vi "GetValuesFromRefs_USB7855R.vi"(6 "Array":cluster{"LSB Weight":u32, "Offset":i32}[](array[cluster]), 11 "ChangeonFly":T2) -> (3 "output cluster":T1)   [LabVIEW 2023]
uses:
  TypeDefs/ChangeOnFly.ctl
  User_Vi/Settings.vi
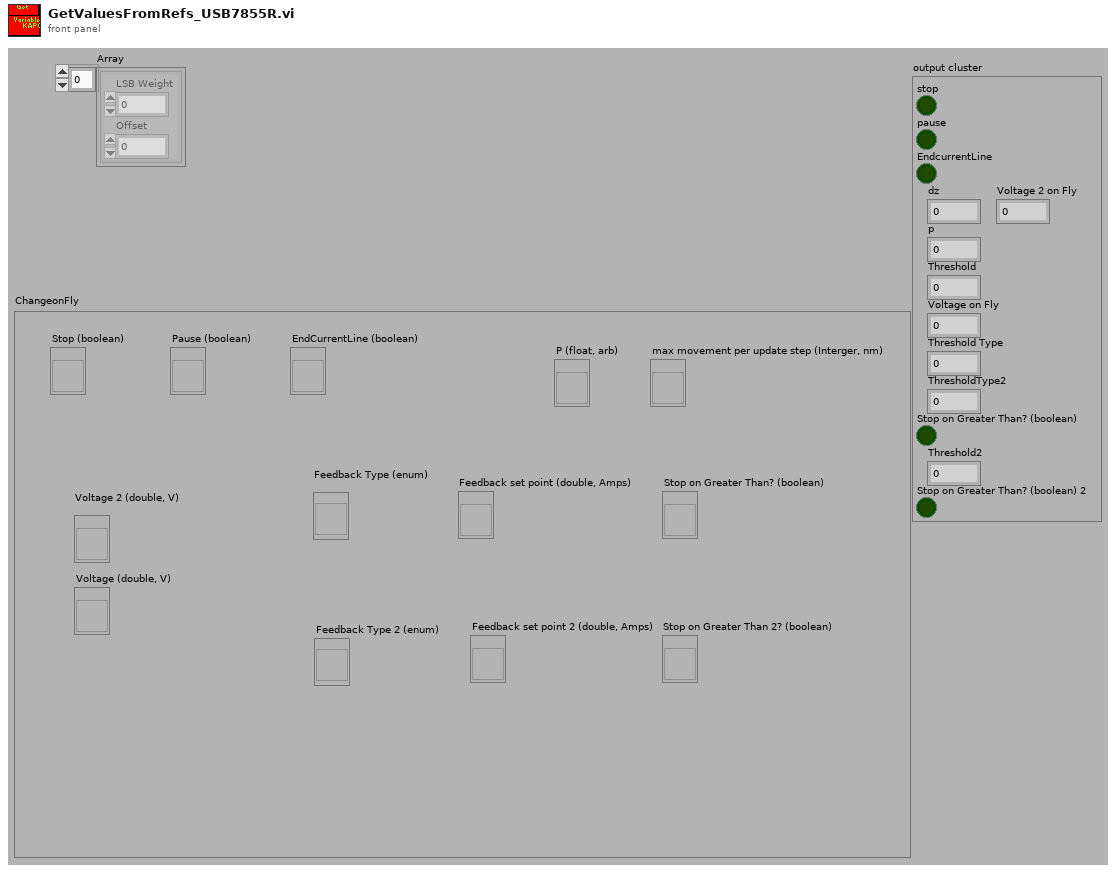
[diagram p1: front panel]
types:
  T1 = cluster{"stop":bool, "pause":bool, "EndcurrentLine":bool, "dz":i32, "p":fxp<+/-,32,1>, "Threshold":i32, "Voltage on Fly":i16, "Threshold Type":u8, "ThresholdType2":u8, "Stop on Greater Than? (boolean)":bool, "Threshold2":i32, "Stop on Greater Than? (boolean) 2":bool, "Voltage 2 on Fly":i16}
  T2 = typedef "ChangeOnFly.ctl" = cluster{"Stop (boolean)":refnum<vi>, "Pause (boolean)":refnum<vi>, "EndCurrentLine (boolean)":refnum<vi>, "max movement per update step (Interger, nm)":refnum<vi>, "P (float, arb)":refnum<vi>, "Feedback set point (double, Amps)":refnum<vi>, "Voltage (double, V)":refnum<vi>, "Feedback set point 2 (double, Amps)":refnum<vi>, "Stop on Greater Than 2? (boolean)":refnum<vi>, "Stop on Greater Than? (boolean)":refnum<vi>, "Voltage 2 (double, V)":refnum<vi>, "Feedback Type (enum)":refnum<vi>, "Feedback Type 2 (enum)":refnum<vi>}
  T3 = enum16{"AC Magnitude", "Current 1", "Current 2", "Phase"}
  T4 = enum16{"USB 7855 (AI)", "USB 7855 (AO)", "USB 7855 OEM (AI)", "USB 7855 OEM (AO)", "USB 7856  (AI)", "USB 7856 (AO)", "USB 7856 OEM (AI)", "USB 7856 OEM (AO)"}
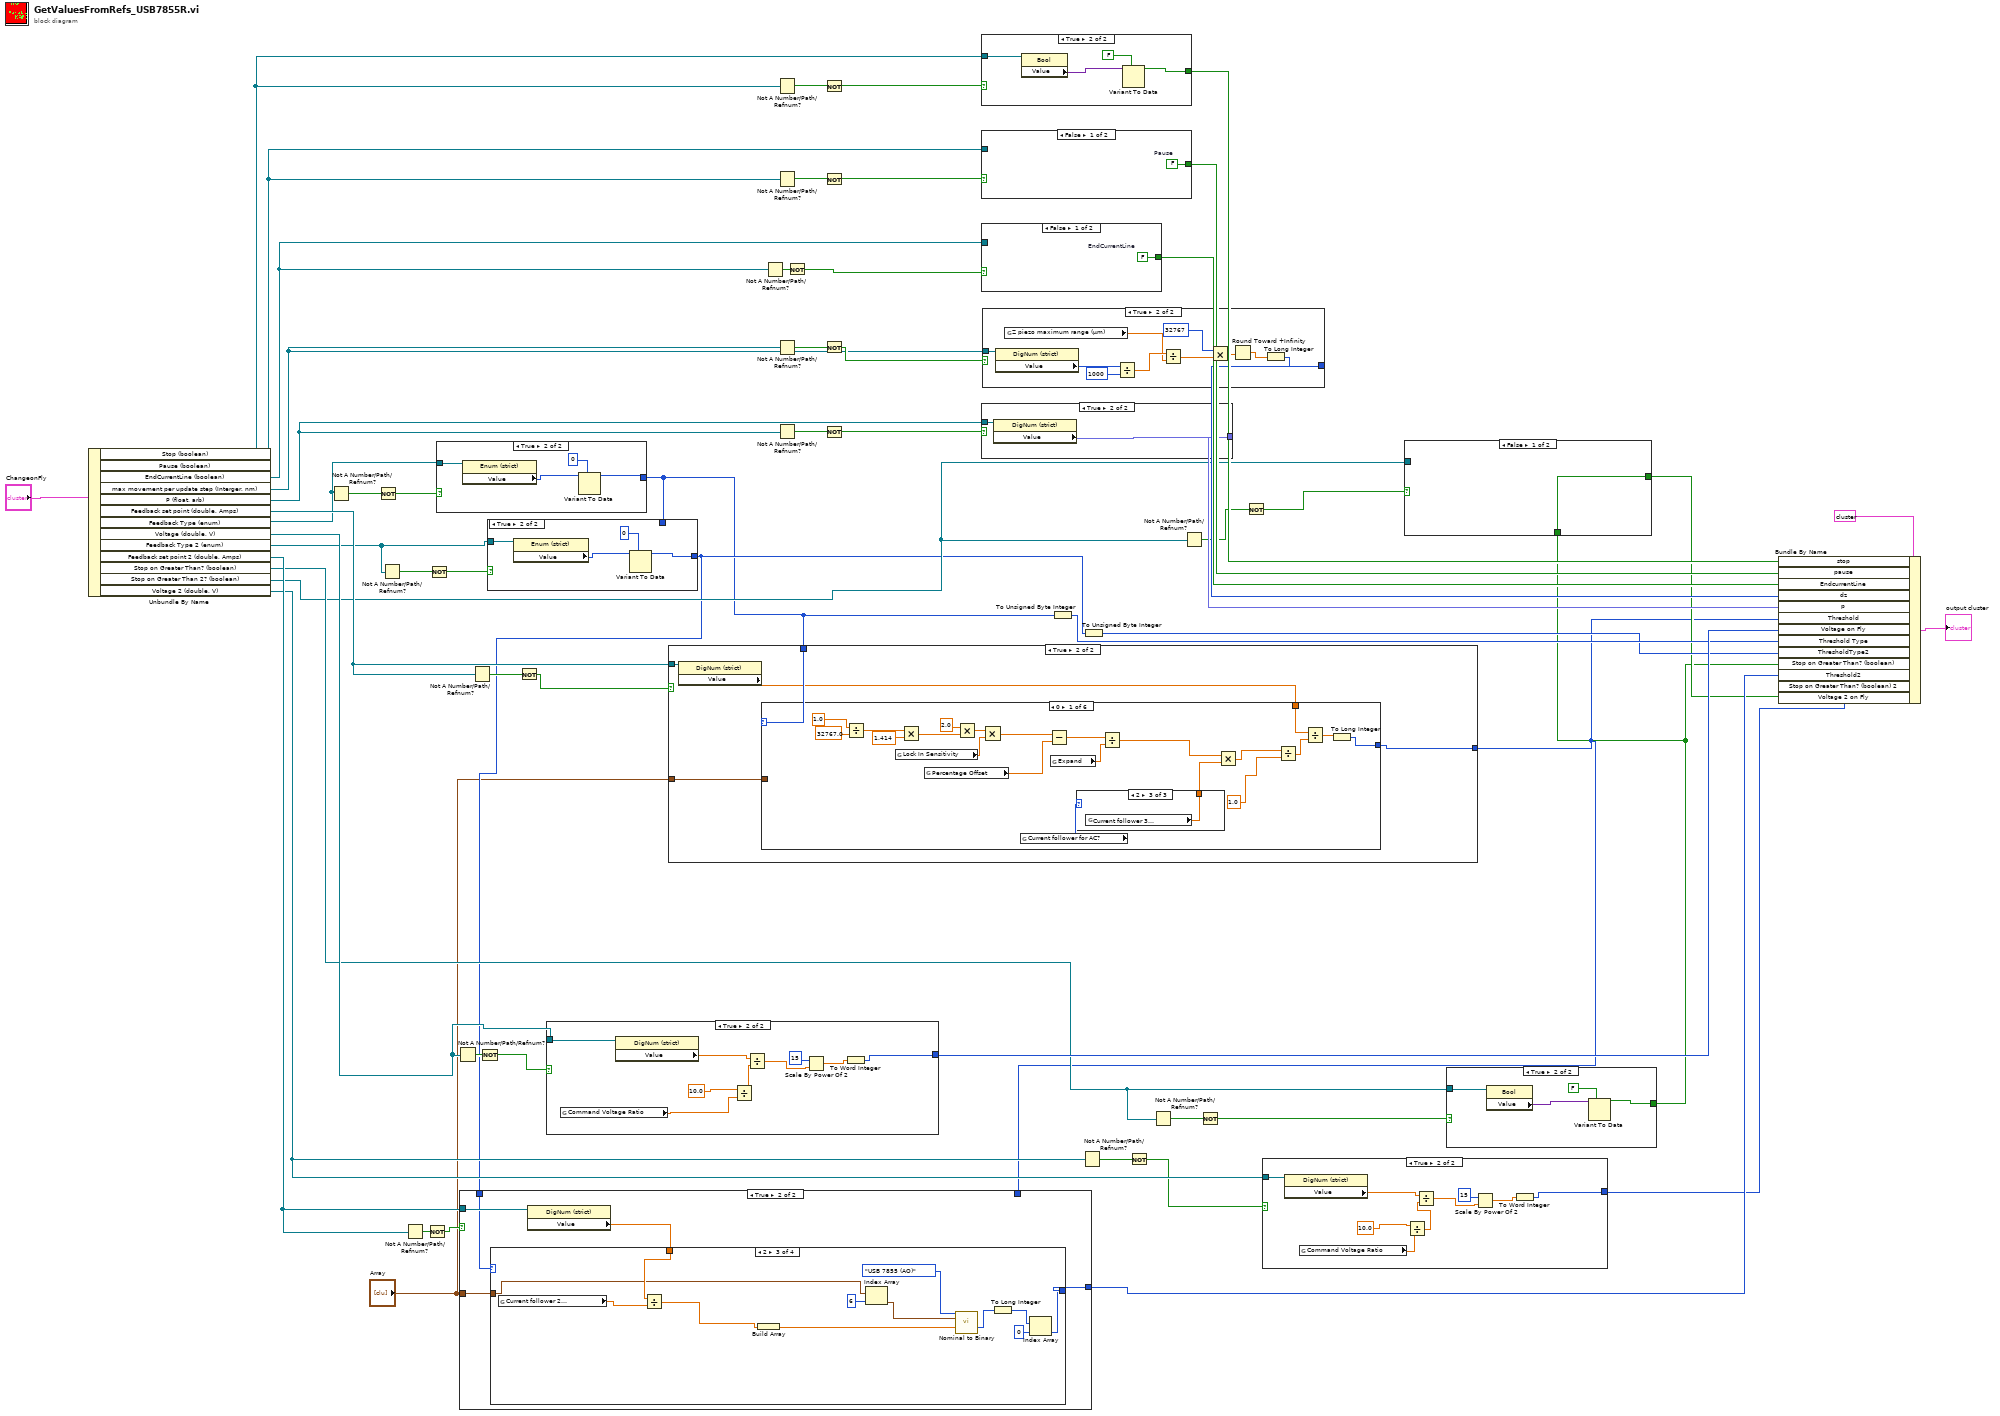
[diagram p0: block diagram]
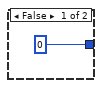
[diagram p3: hidden frame]
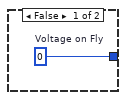
[diagram p4: hidden frame]
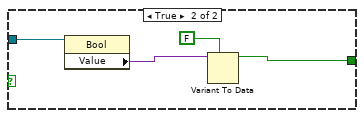
[diagram p5: hidden frame]
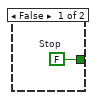
[diagram p6: hidden frame]
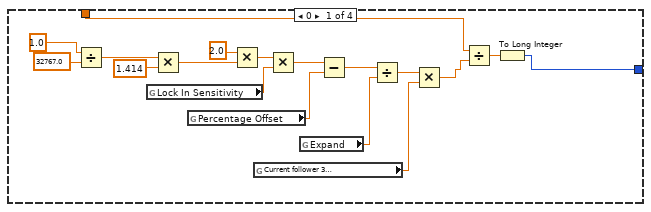
[diagram p8: hidden frame]
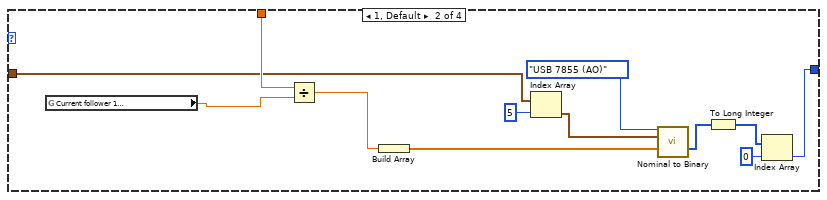
[diagram p9: hidden frame]
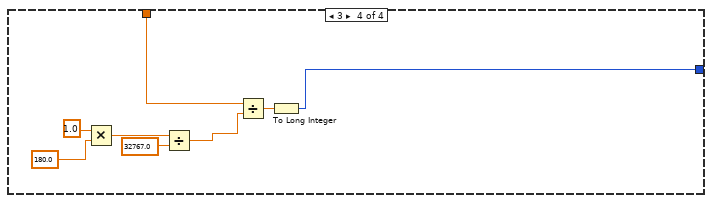
[diagram p10: hidden frame]
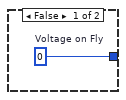
[diagram p11: hidden frame]
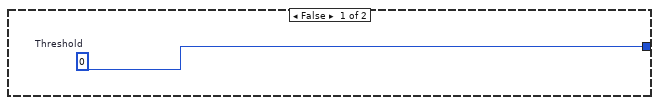
[diagram p12: hidden frame]
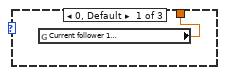
[diagram p13: hidden frame]
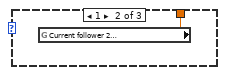
[diagram p14: hidden frame]
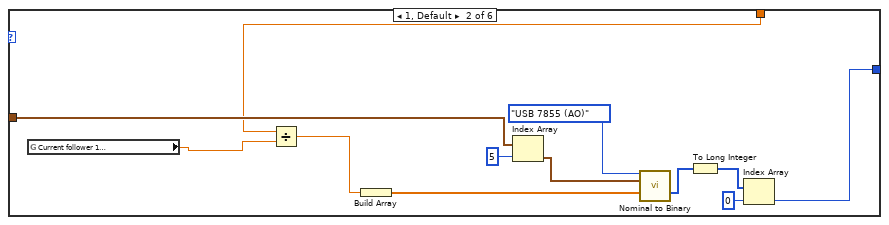
[diagram p15: hidden frame]
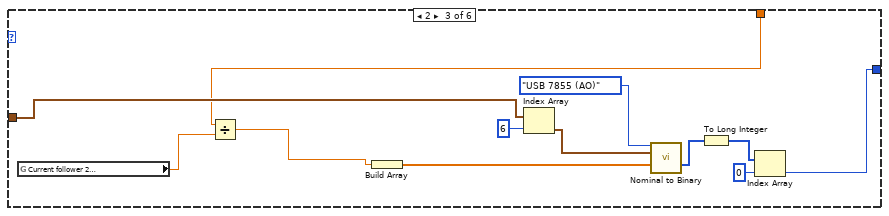
[diagram p16: hidden frame]
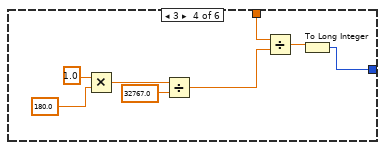
[diagram p17: hidden frame]
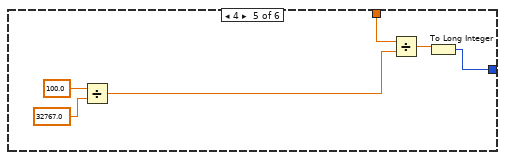
[diagram p18: hidden frame]
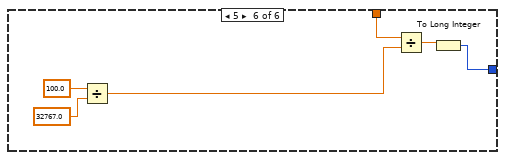
[diagram p19: hidden frame]
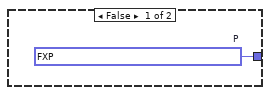
[diagram p20: hidden frame]
diagram:
  n1 = Unbundle By Name("ChangeonFly") -> ("Stop (boolean)"=w12:refnum<vi>, "Pause (boolean)"=w54:refnum<vi>, "EndCurrentLine (boolean)"=w51:refnum<vi>, "max movement per update step (Interger, nm)"=w48:refnum<vi>, "P (float, arb)"=w45:refnum<vi>, "Feedback set point (double, Amps)"=w37:refnum<vi>, "Feedback Type (enum)"=w9:refnum<vi>, "Voltage (double, V)"=w34:refnum<vi>, "Feedback Type 2 (enum)"=w8:refnum<vi>, "Feedback set point 2 (double, Amps)"=w24:refnum<vi>, "Stop on Greater Than? (boolean)"=w21:refnum<vi>, "Stop on Greater Than 2? (boolean)"=w18:refnum<vi>, "Voltage 2 (double, V)"=w14:refnum<vi>)
  n2 = Not A Number/Path/Refnum?(number/path/refnum=w9) -> (NaN/Path/Refnum?=w11:bool)
  n3 = Not(x=w11) -> (.not. x?=w10:bool)
  n4 = Not A Number/Path/Refnum?(number/path/refnum=w8) -> (NaN/Path/Refnum?=w7:bool)
  n5 = Not A Number/Path/Refnum?(number/path/refnum=w24) -> (NaN/Path/Refnum?=w31:bool)
  n6 = Not(x=w31) -> (.not. x?=w30:bool)
  n7 = Not(x=w7) -> (.not. x?=w6:bool)
  n8 = case shown="True" w10 {
    tunnel: w9 -> [_ w62]
    tunnel: [0 ("y") w60] -> w4
    frame False {
    }
    frame True {
      n9 = property on="Property Node" class="Enum (strict)"(reference=w62) -> ("Value"=w63:T3)  [unwired: 1 in, 2 out]
      n10 = Variant To Data(type=0 ("y"), Variant=w63) -> (data=w60:i32)  [unwired: 1 in, 1 out]
    }
  }
  n11 = Not A Number/Path/Refnum?(number/path/refnum=w34) -> (NaN/Path/Refnum?=w36:bool)
  n12 = Not A Number/Path/Refnum?(number/path/refnum=w37) -> (NaN/Path/Refnum?=w44:bool)
  n13 = Not(x=w36) -> (.not. x?=w35:bool)
  n14 = case shown="True" w6 {
    tunnel: [w64 w66] -> w5
    tunnel: w8 -> [_ w67]
    tunnel: w4 -> [w64 _]
    frame False {
    }
    frame True {
      n15 = property on="Property Node" class="Enum (strict)"(reference=w67) -> ("Value"=w68:T3)  [unwired: 1 in, 2 out]
      n16 = Variant To Data(type=0 ("y"), Variant=w68) -> (data=w66:i32)  [unwired: 1 in, 1 out]
    }
  }
  n17 = Not(x=w44) -> (.not. x?=w43:bool)
  n18 = case shown="True" w35 {
    tunnel: [w69 w73] -> w33
    tunnel: w34 -> [_ w78]
    frame False {
      w69 = i16 0  # Voltage on Fly
    }
    frame True {
      n19 = global read "Settings.vi" "Command Voltage Ratio"() -> (w70:dbl)
      n20 = property on="Property Node" class="DigNum (strict)"(reference=w78) -> ("Value"=w77:dbl)  [unwired: 1 in, 2 out]
      n21 = Divide(x=10.0 ("Max/Min Value [V]"), y=w70) -> (x/y=w71:dbl)
      n22 = Divide(x=w77, y=w71) -> (x/y=w75:dbl)
      n23 = Scale By Power Of 2(n=15, x=w75) -> (x*2^n=w74:dbl)
      n24 = To Word Integer(number=w74) -> (16bit integer=w73:i16)
    }
  }
  n25 = case shown="True" w43 {
    tunnel: w37 -> [_ w84]
    tunnel: [w79 w81] -> w3
    tunnel: w4 -> [_ w83]
    tunnel: "Array" -> [_ w80]
    frame False {
      w79 = 0  # Threshold
    }
    frame True {
      n26 = property on="Property Node" class="DigNum (strict)"(reference=w84) -> ("Value"=w82:dbl)  [unwired: 1 in, 2 out]
      n27 = case shown="0" w83 {
        tunnel: [w85 w109 w121 w133 w141 w147] -> w81
        tunnel: w82 -> [w87 w110 w123 w135 w143 w149]
        tunnel: w80 -> [_ w111 w124 _ _ _]
        frame 0 {
          n28 = Divide(x=1.0, y=32767.0 ("n")) -> (x/y=w97:dbl)
          n29 = global read "Settings.vi" "Lock In Sensitivity"() -> (w104:dbl)
          n30 = Multiply(x=w97, y=1.414) -> (x*y=w98:dbl)
          n31 = global read "Settings.vi" "Percentage Offset"() -> (w94:dbl)
          n32 = Multiply(x=2.0 ("y"), y=w98) -> (x*y=w103:dbl)
          n33 = Multiply(x=w103, y=w104) -> (x*y=w105:dbl)
          n34 = global read "Settings.vi" "Current follower for AC?"() -> (w89:u8)
          n35 = Subtract(x=w105, y=w94) -> (x-y=w100:dbl)
          n36 = global read "Settings.vi" "Expand"() -> (w101:dbl)
          n37 = case shown="2" w89 {
            tunnel: [w106 w107 w108] -> w92
            frame 0, Default {
              n38 = global read "Settings.vi" "Current follower 1\n (AI-3)"() -> (w106:dbl)
            }
            frame 1 {
              n39 = global read "Settings.vi" "Current follower 2 \n(AI-4)"() -> (w107:dbl)
            }
            frame 2 {
              n40 = global read "Settings.vi" "Current follower 3\n(AI-6)"() -> (w108:dbl)
            }
          }
          n41 = Divide(x=w100, y=w101) -> (x/y=w102:dbl)
          n42 = Multiply(x=w102, y=w92) -> (x*y=w91:dbl)
          n43 = Divide(x=w91, y=1.0 ("x")) -> (x/y=w86:dbl)
          n44 = Divide(x=w87, y=w86) -> (x/y=w88:dbl)
          n45 = To Long Integer(number=w88) -> (32bit integer=w85:i32)
        }
        frame 1, Default {
          n46 = global read "Settings.vi" "Current follower 1\n (AI-3)"() -> (w114:dbl)
          n47 = Divide(x=w110, y=w114) -> (x/y=w119:dbl)
          n48 = Build Array(w119) -> (w113:dbl[])
          n49 = Index Array(array=w111, index=5) -> (element=w120:cluster{"LSB Weight":u32, "Offset":i32})
          n50 = call "Nominal to Binary.vi"("Target Type"=T4."USB 7855 (AO)", "Calibration"=w120, "Nominal Value"=w113) -> ("Binary Value"=w116:i32[])  [unwired: 12 in]
          n51 = To Long Integer(number=w116) -> (32bit integer=w117:i32[])
          n52 = Index Array(array=w117, index=0) -> (element=w109:i32)
        }
        frame 2 {
          n53 = global read "Settings.vi" "Current follower 2 \n(AI-4)"() -> (w122:dbl)
          n54 = Divide(x=w123, y=w122) -> (x/y=w132:dbl)
          n55 = Build Array(w132) -> (w125:dbl[])
          n56 = Index Array(array=w124, index=6) -> (element=w128:cluster{"LSB Weight":u32, "Offset":i32})
          n57 = call "Nominal to Binary.vi"("Target Type"=T4."USB 7855 (AO)", "Calibration"=w128, "Nominal Value"=w125) -> ("Binary Value"=w126:i32[])  [unwired: 12 in]
          n58 = To Long Integer(number=w126) -> (32bit integer=w127:i32[])
          n59 = Index Array(array=w127, index=0) -> (element=w121:i32)
        }
        frame 3 {
          n60 = Multiply(x=1.0 ("Max Value [um]"), y=180.0 ("Max Value [um]")) -> (x*y=w139:dbl)
          n61 = Divide(x=w139, y=32767.0 ("n")) -> (x/y=w134:dbl)
          n62 = Divide(x=w135, y=w134) -> (x/y=w136:dbl)
          n63 = To Long Integer(number=w136) -> (32bit integer=w133:i32)
        }
        frame 4 {
          n64 = Divide(x=100.0, y=32767.0 ("x")) -> (x/y=w142:dbl)
          n65 = Divide(x=w143, y=w142) -> (x/y=w144:dbl)
          n66 = To Long Integer(number=w144) -> (32bit integer=w141:i32)
        }
        frame 5 {
          n67 = Divide(x=100.0, y=32767.0 ("x")) -> (x/y=w148:dbl)
          n68 = Divide(x=w149, y=w148) -> (x/y=w150:dbl)
          n69 = To Long Integer(number=w150) -> (32bit integer=w147:i32)
        }
      }
    }
  }
  n70 = case shown="True" w30 {
    tunnel: [w153 w155] -> w26
    tunnel: w24 -> [_ w158]
    tunnel: w5 -> [_ w157]
    tunnel: w3 -> [w153 _]
    tunnel: "Array" -> [_ w154]
    frame False {
    }
    frame True {
      n71 = property on="Property Node" class="DigNum (strict)"(reference=w158) -> ("Value"=w156:dbl)  [unwired: 1 in, 2 out]
      n72 = case shown="2" w157 {
        tunnel: [w159 w183 w189 w201] -> w155
        tunnel: w156 -> [w160 w188 w193 w202]
        tunnel: w154 -> [_ w177 w190 _]
        frame 0 {
          n73 = Divide(x=1.0, y=32767.0 ("n")) -> (x/y=w168:dbl)
          n74 = global read "Settings.vi" "Lock In Sensitivity"() -> (w175:dbl)
          n75 = Multiply(x=w168, y=1.414) -> (x*y=w169:dbl)
          n76 = global read "Settings.vi" "Percentage Offset"() -> (w164:dbl)
          n77 = Multiply(x=2.0 ("y"), y=w169) -> (x*y=w174:dbl)
          n78 = global read "Settings.vi" "Current follower 3\n(AI-6)"() -> (w166:dbl)
          n79 = Multiply(x=w174, y=w175) -> (x*y=w176:dbl)
          n80 = global read "Settings.vi" "Expand"() -> (w172:dbl)
          n81 = Subtract(x=w176, y=w164) -> (x-y=w171:dbl)
          n82 = Divide(x=w171, y=w172) -> (x/y=w173:dbl)
          n83 = Multiply(x=w173, y=w166) -> (x*y=w161:dbl)
          n84 = Divide(x=w160, y=w161) -> (x/y=w162:dbl)
          n85 = To Long Integer(number=w162) -> (32bit integer=w159:i32)
        }
        frame 1, Default {
          n86 = global read "Settings.vi" "Current follower 1\n (AI-3)"() -> (w185:dbl)
          n87 = Divide(x=w188, y=w185) -> (x/y=w179:dbl)
          n88 = Build Array(w179) -> (w186:dbl[])
          n89 = Index Array(array=w177, index=5) -> (element=w178:cluster{"LSB Weight":u32, "Offset":i32})
          n90 = call "Nominal to Binary.vi"("Target Type"=T4."USB 7855 (AO)", "Calibration"=w178, "Nominal Value"=w186) -> ("Binary Value"=w182:i32[])  [unwired: 12 in]
          n91 = To Long Integer(number=w182) -> (32bit integer=w181:i32[])
          n92 = Index Array(array=w181, index=0) -> (element=w183:i32)
        }
        frame 2 {
          n93 = global read "Settings.vi" "Current follower 2 \n(AI-4)"() -> (w192:dbl)
          n94 = Divide(x=w193, y=w192) -> (x/y=w191:dbl)
          n95 = Build Array(w191) -> (w200:dbl[])
          n96 = Index Array(array=w190, index=6) -> (element=w197:cluster{"LSB Weight":u32, "Offset":i32})
          n97 = call "Nominal to Binary.vi"("Target Type"=T4."USB 7855 (AO)", "Calibration"=w197, "Nominal Value"=w200) -> ("Binary Value"=w199:i32[])  [unwired: 12 in]
          n98 = To Long Integer(number=w199) -> (32bit integer=w198:i32[])
          n99 = Index Array(array=w198, index=0) -> (element=w189:i32)
        }
        frame 3 {
          n100 = Multiply(x=1.0 ("Max Value [um]"), y=180.0 ("Max Value [um]")) -> (x*y=w207:dbl)
          n101 = Divide(x=w207, y=32767.0 ("n")) -> (x/y=w203:dbl)
          n102 = Divide(x=w202, y=w203) -> (x/y=w204:dbl)
          n103 = To Long Integer(number=w204) -> (32bit integer=w201:i32)
        }
      }
    }
  }
  n104 = Not A Number/Path/Refnum?(number/path/refnum=w51) -> (NaN/Path/Refnum?=w53:bool)
  n105 = Not A Number/Path/Refnum?(number/path/refnum=w12) -> (NaN/Path/Refnum?=w58:bool)
  n106 = Not A Number/Path/Refnum?(number/path/refnum=w54) -> (NaN/Path/Refnum?=w55:bool)
  n107 = Not A Number/Path/Refnum?(number/path/refnum=w48) -> (NaN/Path/Refnum?=w49:bool)
  n108 = Not A Number/Path/Refnum?(number/path/refnum=w45) -> (NaN/Path/Refnum?=w47:bool)
  n109 = Not(x=w53) -> (.not. x?=w52:bool)
  n110 = Not(x=w58) -> (.not. x?=w57:bool)
  n111 = Not(x=w55) -> (.not. x?=w56:bool)
  n112 = Not(x=w49) -> (.not. x?=w50:bool)
  n113 = Not(x=w47) -> (.not. x?=w46:bool)
  n114 = case shown="True" w57 {
    tunnel: [w209 w210] -> w42
    tunnel: w12 -> [_ w211]
    frame False {
      w209 = FALSE  # Stop
    }
    frame True {
      n115 = property on="Property Node" class="Bool"(reference=w211) -> ("Value"=w213:variant)  [unwired: 1 in, 2 out]
      n116 = Variant To Data(type=FALSE ("stop"), Variant=w213) -> (data=w210:bool)  [unwired: 1 in, 1 out]
    }
  }
  n117 = case shown="False" w56 {
    tunnel: [w214 w215] -> w41
    tunnel: w54 -> [_ w216]
    frame False {
      w214 = FALSE  # Pause
    }
    frame True {
      n118 = property on="Property Node" class="Bool"(reference=w216) -> ("Value"=w218:variant)  [unwired: 1 in, 2 out]
      n119 = Variant To Data(type=FALSE ("stop"), Variant=w218) -> (data=w215:bool)  [unwired: 1 in, 1 out]
    }
  }
  n120 = case shown="False" w52 {
    tunnel: [w219 w220] -> w40
    tunnel: w51 -> [_ w221]
    frame False {
      w219 = FALSE  # EndCurrentLine
    }
    frame True {
      n121 = property on="Property Node" class="Bool"(reference=w221) -> ("Value"=w223:variant)  [unwired: 1 in, 2 out]
      n122 = Variant To Data(type=FALSE ("stop"), Variant=w223) -> (data=w220:bool)  [unwired: 1 in, 1 out]
    }
  }
  n123 = case shown="True" w46 {
    tunnel: w45 -> [_ w226]
    tunnel: [w224 w225] -> w38
    frame False {
      w224 = fxp<+/-,32,1> 0.0  # P
    }
    frame True {
      n124 = property on="Property Node" class="DigNum (strict)"(reference=w226) -> ("Value"=w225:fxp<+/-,32,1>)  [unwired: 1 in, 2 out]
    }
  }
  n125 = case shown="True" w50 {
    tunnel: w48 -> [_ w237]
    tunnel: [w227 w228] -> w39
    frame False {
      w227 = 0  # UpperdZ
    }
    frame True {
      n126 = property on="Property Node" class="DigNum (strict)"(reference=w237) -> ("Value"=w236:i32)  [unwired: 1 in, 2 out]
      n127 = global read "Settings.vi" "Z piezo maximum range (µm)"() -> (w233:dbl)
      n128 = Divide(x=w236, y=1000) -> (x/y=w234:dbl)
      n129 = Divide(x=w234, y=w233) -> (x/y=w232:dbl)
      n130 = Multiply(x=i16 32767, y=w232) -> (x*y=w230:dbl)
      n131 = Round Toward +Infinity(x=w230) -> (ceil(x): smallest int >= x=w229:dbl)
      n132 = To Long Integer(number=w229) -> (32bit integer=w228:i32)
    }
  }
  n133 = To Unsigned Byte Integer(number=w4) -> (unsigned 8bit integer=w28:u8)
  n134 = Not A Number/Path/Refnum?(number/path/refnum=w14) -> (NaN/Path/Refnum?=w15:bool)
  n135 = To Unsigned Byte Integer(number=w5) -> (unsigned 8bit integer=w27:u8)
  n136 = Not(x=w15) -> (.not. x?=w13:bool)
  n137 = Not A Number/Path/Refnum?(number/path/refnum=w21) -> (NaN/Path/Refnum?=w22:bool)
  n138 = Not A Number/Path/Refnum?(number/path/refnum=w18) -> (NaN/Path/Refnum?=w20:bool)
  n139 = Not(x=w22) -> (.not. x?=w23:bool)
  n140 = Not(x=w20) -> (.not. x?=w19:bool)
  n141 = case shown="True" w13 {
    tunnel: [w238 w242] -> w16
    tunnel: w14 -> [_ w247]
    frame False {
      w238 = i16 0  # Voltage on Fly
    }
    frame True {
      n142 = property on="Property Node" class="DigNum (strict)"(reference=w247) -> ("Value"=w246:dbl)  [unwired: 1 in, 2 out]
      n143 = global read "Settings.vi" "Command Voltage Ratio"() -> (w241:dbl)
      n144 = Divide(x=10.0 ("Max/Min Value [V]"), y=w241) -> (x/y=w239:dbl)
      n145 = Divide(x=w246, y=w239) -> (x/y=w244:dbl)
      n146 = Scale By Power Of 2(n=15, x=w244) -> (x*2^n=w243:dbl)
      n147 = To Word Integer(number=w243) -> (16bit integer=w242:i16)
    }
  }
  n148 = case shown="True" w23 {
    tunnel: [w248 w249] -> w2
    tunnel: w21 -> [_ w250]
    frame False {
      w248 = FALSE  # Stop
    }
    frame True {
      n149 = property on="Property Node" class="Bool"(reference=w250) -> ("Value"=w252:variant)  [unwired: 1 in, 2 out]
      n150 = Variant To Data(type=FALSE ("stop"), Variant=w252) -> (data=w249:bool)  [unwired: 1 in, 1 out]
    }
  }
  n151 = case shown="False" w19 {
    tunnel: [w253 w254] -> w17
    tunnel: w18 -> [_ w255]
    tunnel: w2 -> [w253 _]
    frame False {
    }
    frame True {
      n152 = property on="Property Node" class="Bool"(reference=w255) -> ("Value"=w257:variant)  [unwired: 1 in, 2 out]
      n153 = Variant To Data(type=FALSE ("stop"), Variant=w257) -> (data=w254:bool)  [unwired: 1 in, 1 out]
    }
  }
  n154 = Bundle By Name(cluster=T1 {"stop"=FALSE, "pause"=FALSE, "EndcurrentLine"=FALSE, "dz"=0, "p"=0.0, "Threshold"=0, "Voltage on Fly"=0, "Threshold Type"=0, "ThresholdType2"=0, "Stop on Greater Than? (boolean)"=FALSE, "Threshold2"=0, "Stop on Greater Than? (boolean) 2"=FALSE, "Voltage 2 on Fly"=0} ("input cluster"), "stop"=w42, "pause"=w41, "EndcurrentLine"=w40, "dz"=w39, "p"=w38, "Threshold"=w3, "Voltage on Fly"=w33, "Threshold Type"=w28, "ThresholdType2"=w27, "Stop on Greater Than? (boolean)"=w2, "Threshold2"=w26, "Stop on Greater Than? (boolean) 2"=w17, "Voltage 2 on Fly"=w16) -> (→"output cluster":T1)
